vi "TL error.vi"(7 "Input string":string, 8 "error in (no error)":errorcluster, 9 "Serial number of motor":string, 11 "Return Code":i32) -> (0 "error out":errorcluster)   [LabVIEW 2014]
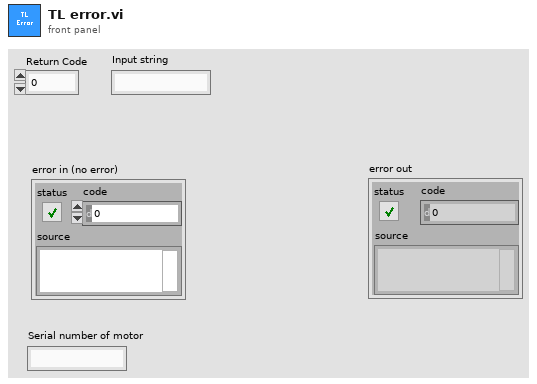
[diagram p1: front panel]
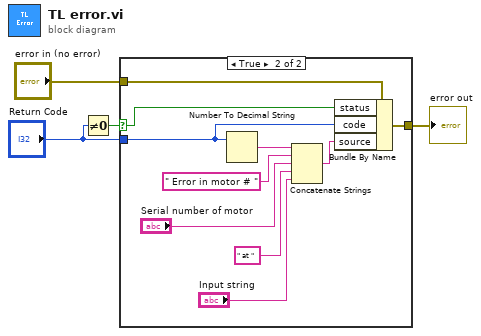
[diagram p0: block diagram]
diagram:
  n1 = Not Equal To 0?(x="Return Code") -> (x != 0?=w3:bool)
  n2 = case shown="True" w3 {
    selector: w3 -> [_ w14]
    tunnel: "Return Code" -> [_ w9]
    tunnel: "error in (no error)" -> [w5 w15]
    tunnel: [w5 w13] -> w1
    frame False {
    }
    frame True {
      n3 = Number To Decimal String(number=w9) -> (decimal integer string=w8:string)  [unwired: 1 in]
      n4 = Concatenate Strings(w8, " Error in motor # ", "Serial number of motor", " at ", "Input string") -> (w10:string)
      n5 = Bundle By Name(cluster=w15, "status"=w14, "code"=w9, "source"=w10) -> (w13:errorcluster)
    }
  }
  "error out" <- w1
